vi "Dashboard.vi"   [LabVIEW 2016]
uses:
  Drive/Drive Globals.vi
  Rotation/Rotation Globals.vi
  <vilib>/Rock Robotics/Network Tables/NT Write Numeric Array.vi
  <vilib>/Rock Robotics/Network Tables/NT Write Boolean.vi
  <vilib>/Rock Robotics/Network Tables/NT Write String.vi
types:
  T1 = typedef "Drive Notifier.ctl" = cluster{"Parameter 1":dbl, "Parameter 2":dbl, "Parameter 3":dbl, "Drive Control List":T2, "Parameter 4":dbl, "Gear Angle":dbl, "Parameter 6":dbl, "Parameter 7":dbl, "Parameter 8":dbl, "Parameter 9":dbl, "Robotcentric":bool, "Reset Gyro":bool, "Reset Wheels":bool, "Turn to Gear Left":bool, "Turn to Gear Center":bool, "Turn to Gear Right":bool, "Half Power":bool}
  T2 = typedef "Drive Control Type.ctl" = enum16{"No Op", "Fieldcentric", "Robotcentric", "Reset Wheel Position", "Reset Gyro Value", "Turn to Angle", "Drive For Time"}
  T3 = typedef "Rotation Notifier.ctl" = cluster{"Up":bool, "Down":bool, "Rotation Control List":T4, "Control Down":bool, "Manual":bool, "Parameter 1":dbl, "Parameter 2":dbl}
  T4 = typedef "Rotation Control Type.ctl" = enum16{"No Op", "Up", "Down", "Control Up", "Control Down"}
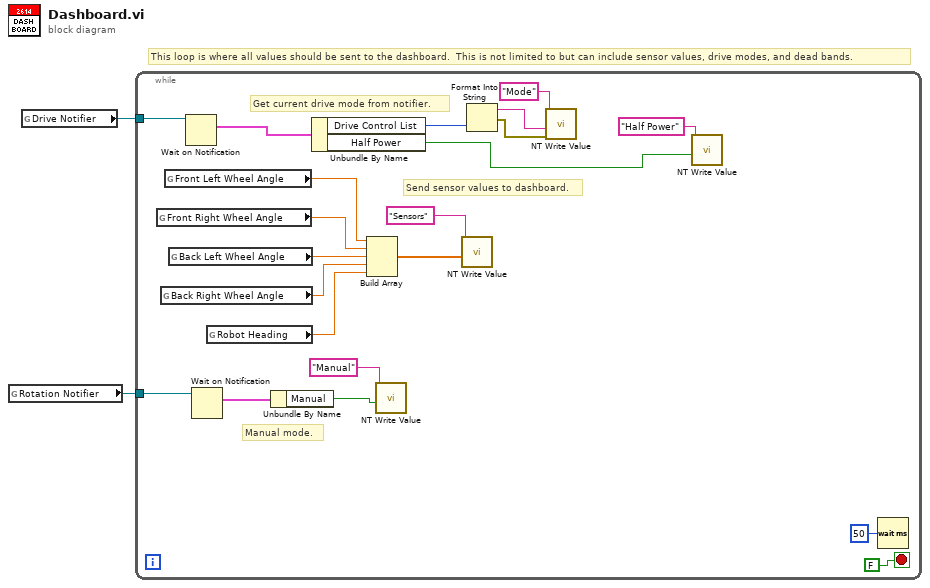
[diagram p0: block diagram]
diagram:
  # "This loop is where all values should be sent to the dashboard.  This is not limited to but can include sensor values, drive modes, and dead bands."
  n1 = global read "Rotation Globals.vi" "Rotation Notifier"() -> (w1:refnum<notifier>)
  n2 = global read "Drive Globals.vi" "Drive Notifier"() -> (w2:refnum<notifier>)
  n3 = while {
    tunnel: w2 -> [w20]
    tunnel: w1 -> [w7]
    stop <- FALSE stop-if-true
    # "Manual mode."
    # "Send sensor values to dashboard."
    # "Get current drive mode from notifier."
    n4 = global read "Drive Globals.vi" "Front Right Wheel Angle"() -> (w14:dbl)
    n5 = global read "Drive Globals.vi" "Back Right Wheel Angle"() -> (w12:dbl)
    n6 = global read "Drive Globals.vi" "Front Left Wheel Angle"() -> (w15:dbl)
    n7 = global read "Drive Globals.vi" "Back Left Wheel Angle"() -> (w13:dbl)
    n8 = Wait on Notification(notifier=w20) -> (notification=w21:T1)  [unwired: 3 in, 3 out]
    n9 = Wait on Notification(notifier=w7) -> (notification=w8:T3)  [unwired: 3 in, 3 out]
    n10 = global read "Drive Globals.vi" "Robot Heading"() -> (w11:dbl)
    n11 = Unbundle By Name(w8) -> ("Manual"=w6:bool)
    n12 = Unbundle By Name(w21) -> ("Drive Control List"=w19:T2, "Half Power"=w3:bool)
    n13 = Build Array(w15, w14, w13, w12, w11) -> (w10:dbl[])
    n14 = call-poly <vilib>:"NT Write Value.vi"("Boolean"=w6, "Name"="Manual") -> ()  [unwired: 9 in, 1 out]
    n15 = call-poly <vilib>:"NT Write Value.vi"("Numeric Array"=w10, "Name"="Sensors") -> ()  [unwired: 9 in, 1 out]
    n16 = Format Into String(w19) -> (resulting string=w17:string, error out=w18:errorcluster)  [unwired: 3 in]
    n17 = call-poly <vilib>:"NT Write Value.vi"("error in"=w18, "String"=w17, "Name"="Mode") -> ()  [unwired: 8 in, 1 out]
    n18 = call-poly <vilib>:"NT Write Value.vi"("Boolean"=w3, "Name"="Half Power") -> ()  [unwired: 9 in, 1 out]
    n19 = Wait (ms)(milliseconds to wait=u32 50) -> ()  [unwired: 1 out]
  }
